vi "Initiate Multipart Upload.vi"(7 "Request Parameters":T2={"Content Type"="binary/octet-stream", "ACL"=enum."private", "Storage Class"=enum."STANDARD", "User Metadata"=[]}, 8 "error in (no error)":errorcluster, 9 "Bucket":string, 10 "Path":string) -> (0 "error out":errorcluster, 3 "Multipart Upload RefNum":T1)   [LabVIEW 2011, in "LV Interface for Amazon S3.lvlib"]
doc: "This operation <B>initiates a multipart upload</B> operation and <B>returns a Multipart Upload Refnum</B>. <B>After</B> initiating a multipart upload process, <B>you can start uploading the individual parts</B> of the object. Multipart uploads provide the following advantages: <B> - Improved throughput</B>: You can upload parts in parallel to improve throughput. <B> - Quick recovery from any network issues</B>: Smaller part size minimizes the impact of restarting a failed upload due to a network error. <B> - Pause and resume object uploads</B>: You can upload object parts over time. Once you initiate a multipart upload there is no expiry; you must explicitly complete or abort the multipart upload. <B> - Begin an upload before you know the final object size</B>: You can upload an object as you are creating it."
uses:
  LV Interface for Amazon S3.lvlib
  Typedefs/AMZ_S3_API_POST Multipart Object Request Parameters.ctl
  Typedefs/AMZ_S3_ACL.ctl
  Typedefs/AMZ_S3_Storage Class.ctl
  Typedefs/AMZ_S3_Object Metadata.ctl
  Typedefs/AMZ_S3_Multipart Upload RefNum.ctl
  Typedefs/AMZ_S3_Multipart Upload RefNum Enum.ctl
  Typedefs/AMZ_S3_Multipart Upload Data.ctl
  Typedefs/AMZ_S3_Multipart Upload Part Data.ctl
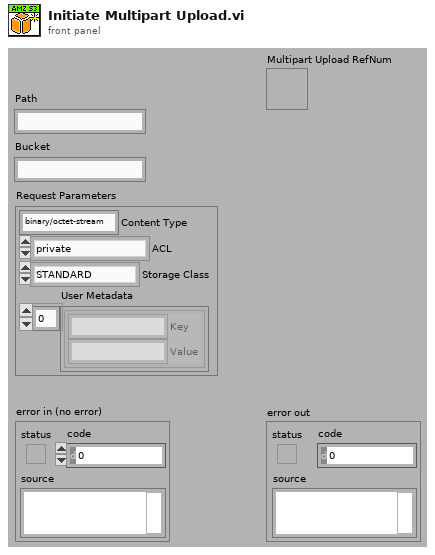
[diagram p1: front panel]
types:
  T1 = typedef "LV Interface for Amazon S3.lvlib/AMZ_S3_Multipart Upload RefNum.ctl" = refnum<k1>
  T2 = typedef "LV Interface for Amazon S3.lvlib/AMZ_S3_API_POST Multipart Object Request Parameters.ctl" = cluster{"Content Type":string, "ACL":T3, "Storage Class":T4, "User Metadata":T5[]}
  T3 = typedef "LV Interface for Amazon S3.lvlib/AMZ_S3_ACL.ctl" = enum16{"private", "public-read", "public-read-write", "authenticated-read", "bucket-owner-read", "bucket-owner-full-control"}
  T4 = typedef "LV Interface for Amazon S3.lvlib/AMZ_S3_Storage Class.ctl" = enum16{"STANDARD", "REDUCED_REDUNDANCY"}
  T5 = typedef "LV Interface for Amazon S3.lvlib/AMZ_S3_Object Metadata.ctl" = cluster{"Key":string, "Value":string}
  T6 = typedef "LV Interface for Amazon S3.lvlib/AMZ_S3_HTTP Header-Value pair.ctl" = cluster{"Header":string, "Value":string}
  T7 = typedef "LV Interface for Amazon S3.lvlib/AMZ_S3_Call Results.ctl" = enum16{"Success", "UndefinedError", "AccessDenied", "AccountProblem", "AmbiguousGrantByEmailAddress", "BadDigest", "BucketAlreadyExists", "BucketAlreadyOwnedByYou", "BucketNotEmpty", "CredentialsNotSupported", "CrossLocationLoggingProhibited", "EntityTooSmall", "EntityTooLarge", "ExpiredToken", "IllegalVersioningConfigurationException", "IncompleteBody", "IncorrectNumberOfFilesInPostRequest", "InlineDataTooLarge", "InternalError", "InvalidAccessKeyId", "InvalidAddressingHeader", "InvalidArgument", "InvalidBucketName", "InvalidDigest", "InvalidLocationConstraint", "InvalidPart", "InvalidPartOrder", "InvalidPayer", "InvalidPolicyDocument", "InvalidRange", "InvalidSecurity", "InvalidSOAPRequest", "InvalidStorageClass", "InvalidTargetBucketForLogging", "InvalidToken", "InvalidURI", "KeyTooLong", "MalformedACLError", "MalformedPOSTRequest", "MalformedXML", "MaxMessageLengthExceeded", "MaxPostPreDataLengthExceededError", "MetadataTooLarge", "MethodNotAllowed", "MissingAttachment", "MissingContentLength", "MissingRequestBodyError", "MissingSecurityElement", "MissingSecurityHeader", "NoLoggingStatusForKey", "NoSuchBucket", "NoSuchKey", "NoSuchUpload", "NoSuchVersion", "NotImplemented", "NotSignedUp", "OperationAborted", "PermanentRedirect", "PreconditionFailed", "Redirect", "RequestIsNotMultiPartContent", "RequestTimeout", "RequestTimeTooSkewed", "RequestTorrentOfBucketError", "SignatureDoesNotMatch", "SlowDown", "TemporaryRedirect", "TokenRefreshRequired", "TooManyBuckets", "UnexpectedContent", "UnresolvableGrantByEmailAddress", "UserKeyMustBeSpecified", "LabVIEWError"}
  T8 = typedef "LV Interface for Amazon S3.lvlib/AMZ_S3_Multipart Upload Data.ctl" = cluster{"Object":string, "Bucket":string, "UploadID":string, "Parts":T9[]}
  T9 = typedef "LV Interface for Amazon S3.lvlib/AMZ_S3_Multipart Upload Part Data.ctl" = cluster{"PartNumber":u16, "Lat modified":timestamp, "ETag":string, "Size":u64}
  T10 = typedef "LV Interface for Amazon S3.lvlib/AMZ_S3_API_InitiateMultipartUploadResult.ctl" = cluster{"Bucket":string, "Key":string, "UploadID":string}
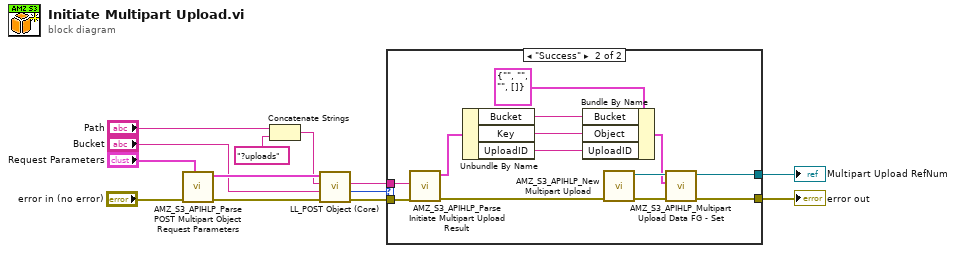
[diagram p0: block diagram]
diagram:
  n1 = call "AMZ_S3_APIHLP_Parse POST Multipart Object Request Parameters.vi"("POST Multipart Object Request Parameters"="Request Parameters", "error in (no error)"="error in (no error)") -> ("error out"=w13:errorcluster, "HTTP Headers"=w12:T6[])  [unwired: 8 in]
  n2 = Concatenate Strings("Path", "?uploads" ("string")) -> (w3:string)
  n3 = call "LL_POST Object (Core).vi"("error in (no error)"=w13, "Bucket"="Bucket", "Path"=w3, "Headers"=w12) -> ("error out"=w7:errorcluster, "Call Result"=w8:T7, "Response body"=w1:string)  [unwired: 4 in, 1 out]
  n4 = case shown="\"Success\"" w8 {
    tunnel: w7 -> [w14 w27]
    tunnel: [w14 w17] -> w6
    tunnel: [_ w16] -> w2
    tunnel: w1 -> [_ w15]
    frame Default {
    }
    frame "Success" {
      n5 = call "AMZ_S3_APIHLP_Parse Initiate Multipart Upload Result.vi"("error in (no error)"=w27, "Response body"=w15) -> ("error out"=w26:errorcluster, "InitiateMultipartUploadResult"=w23:T10)  [unwired: 8 in]
      n6 = Unbundle By Name(w23) -> ("Bucket"=w20:string, "Key"=w21:string, "UploadID"=w19:string)
      n7 = Bundle By Name(cluster=T8 {"Object"="", "Bucket"="", "UploadID"="", "Parts"=[]} ("Multipart Upload Data"), "Bucket"=w20, "Object"=w21, "UploadID"=w19) -> (w18:T8)
      n8 = call "AMZ_S3_APIHLP_New Multipart Upload.vi"("error in (no error)"=w26) -> ("error out"=w25:errorcluster, "Multipart Upload RefNum"=w24:T1)  [unwired: 9 in]
      n9 = call "AMZ_S3_APIHLP_Multipart Upload Data FG - Set.vi"("error in (no error)"=w25, "Multipart Upload Data"=w18, "Multipart Upload RefNum in"=w24) -> ("error out"=w17:errorcluster, "Multipart Upload RefNum out"=w16:T1)  [unwired: 6 in, 1 out]
    }
  }
  "error out" <- w6
  "Multipart Upload RefNum" <- w2
